vi "Open Data RW Results Dialog.vi"(8 "error in (no error)":errorcluster, 9 "Full Element Name":string[](array[string]), 10 "Owning VI Details":T1) -> (0 "error out":errorcluster)   [LabVIEW 2020]
uses:
  synchronization/synchronization.lvclass
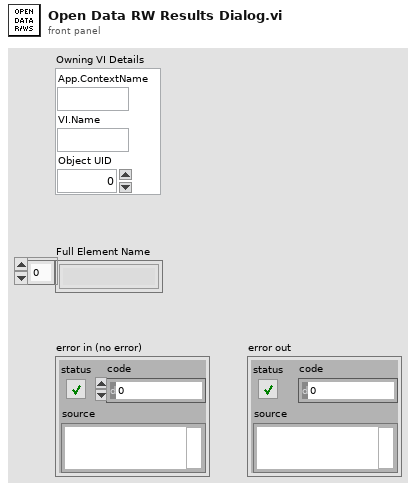
[diagram p1: front panel]
types:
  T1 = cluster{"App.ContextName":string, "VI.Name":string, "Object UID":i32}
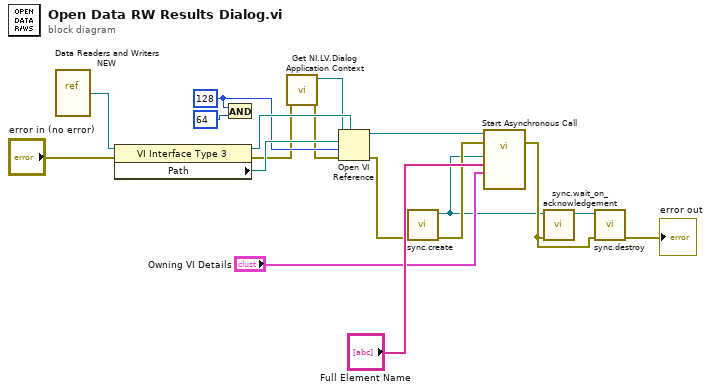
[diagram p0: block diagram]
diagram:
  w12 = 128 ("options")
  n1 = vi-ref "Data Readers and Writers NEW.vi"() -> (w18:refnum<vi>)
  n2 = property class="VI Interface Type 3"(reference=w18, error in="error in (no error)") -> (reference out=w14:refnum<vi>, error out=w10:errorcluster, "Path"=w17:path)
  n3 = And(x=w12, y=64 ("options")) -> ()  [unwired: 1 out]
  n4 = call "Get NI.LV.Dialog Application Context.vi"("error in (no error)"=w10) -> ("error out"=w9:errorcluster, "Application out"=w8:refnum<vi>)  [unwired: 9 in]
  n5 = Open VI Reference(type specifier VI Refnum (for type only)=w14, application reference (local)=w8, vi path=w17, options=w12, error in (no error)=w9) -> (vi reference=w15:refnum<vi>, error out=w5:errorcluster)  [unwired: 1 out]
  n6 = call "sync.create.vi"("error in (no error)"=w5) -> ("error out"=w4:errorcluster, "synchronization"=w1:refnum<class "synchronization.lvclass">)  [unwired: 9 in]
  n7 = call-by-ref "Start Asynchronous Call"(reference=w15, error in=w4, "Owning VI Details"="Owning VI Details", "Full Element Name"="Full Element Name", "synchronization"=w1) -> (error out=w2:errorcluster)  [unwired: 8 in, 2 out]
  n8 = call "sync.wait_on_acknowledgement.vi"("error in (no error)"=w2, "synchronization in"=w1) -> ("synchronization out"=w6:refnum<class "synchronization.lvclass">)  [unwired: 8 in, 1 out]
  n9 = call "sync.destroy.vi"("error in (no error)"=w2, "synchronization"=w6) -> ("error out"=→"error out":errorcluster)  [unwired: 9 in]
